vi "ReadPAQtags.vi"(8 "error in (no error)":errorcluster, 11 "DBAL-BIN in":refnum<class "DBAL-BIN.lvclass">) -> (0 "error out":errorcluster, 2 "PAQ_TAGs":T1 {"TAGprop"."TagFunc" format="%08x"; "TAGprop"."RangeL" format="%.2f"; "TAGprop"."RangeH" format="%.2f"}, 3 "DBAL-BIN out":refnum<class "DBAL-BIN.lvclass">)   [LabVIEW 2020, in "DBAL-BIN.lvclass"]
doc: "Read the PAQ Qtype TAG properties from the database"
uses:
  DBAL-BIN.lvclass
  controls/DBAL_TAGprops.ctl
  controls/DBAL_TAGpropEdit.ctl
  Common/controls/typedef_com_TagProp.ctl
  DBAL-BIN.lvclass/DBAL-BIN.ctl
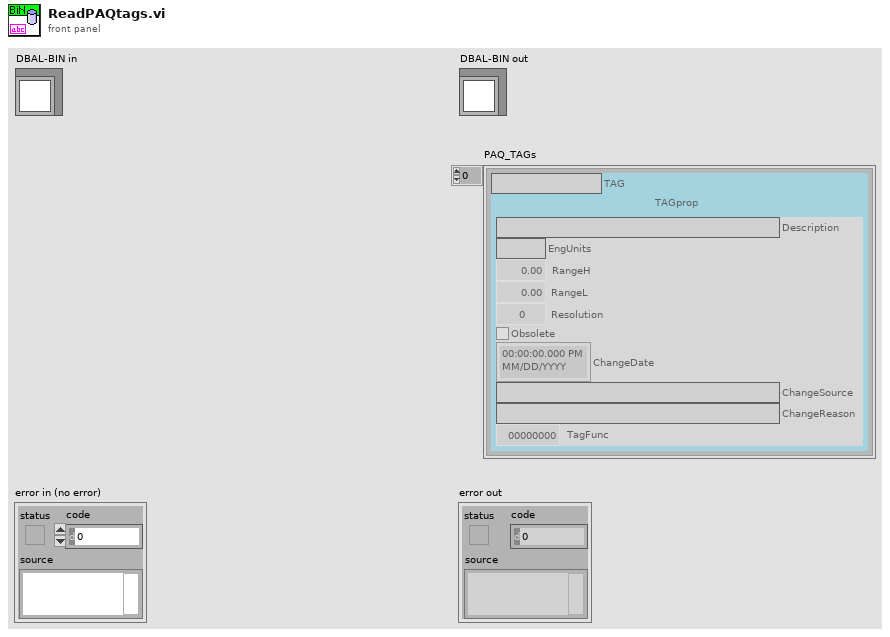
[diagram p1: front panel]
types:
  T1 = typedef "DBAL_TAGprops.ctl" = T2[]
  T2 = typedef "DBAL_TAGpropEdit.ctl" = cluster{"TAG":string, "TAGprop":T3}
  T3 = typedef "typedef_com_TagProp.ctl" = cluster{"Description":string, "EngUnits":string, "RangeH":dbl, "RangeL":dbl, "Resolution":i32, "Obsolete":bool, "ChangeDate":timestamp, "ChangeSource":string, "ChangeReason":string, "TagFunc":u32}
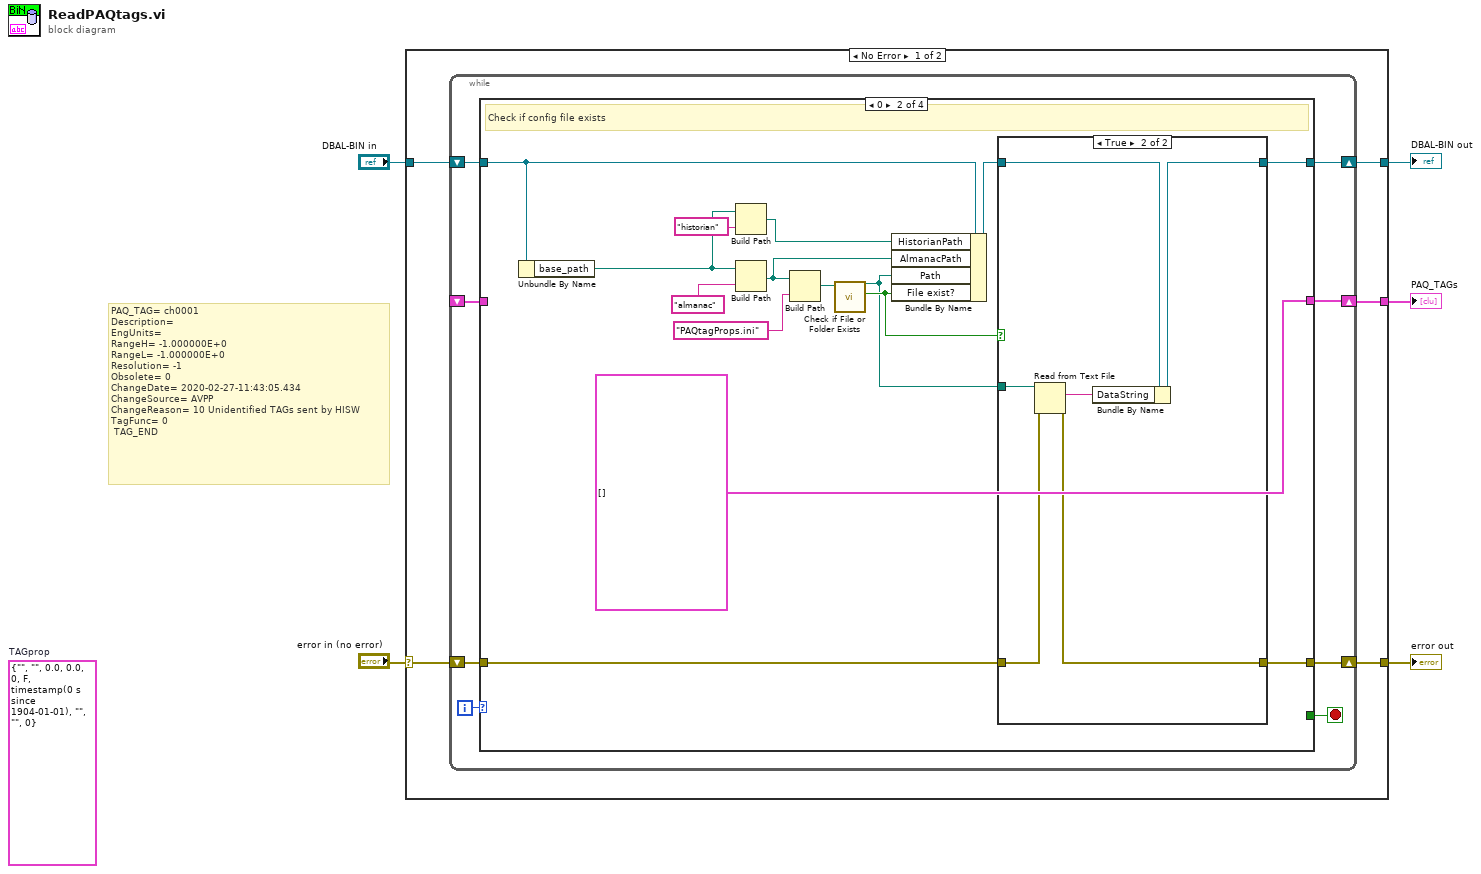
[diagram p0: block diagram]
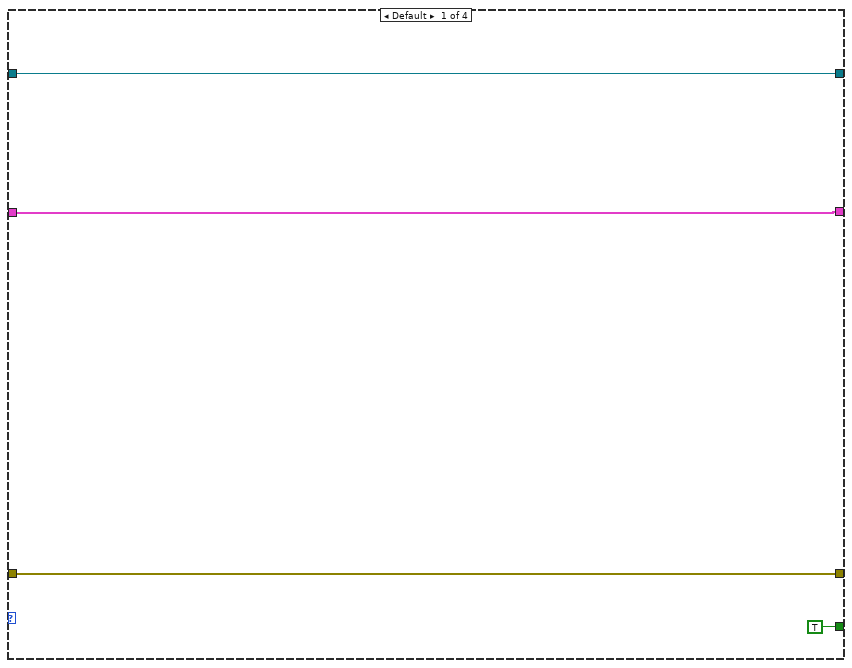
[diagram p2: hidden frame]
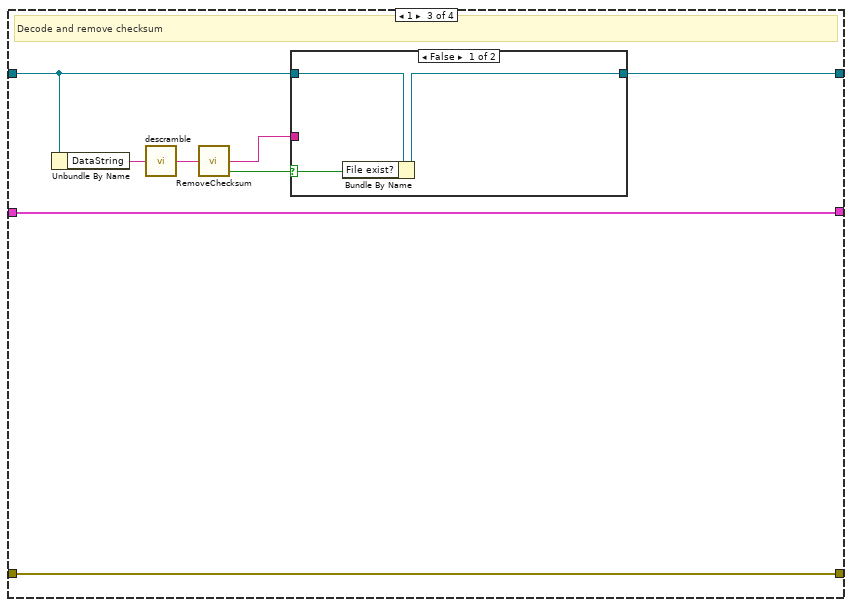
[diagram p4: hidden frame]
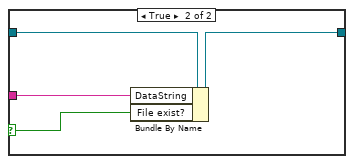
[diagram p5: hidden frame]
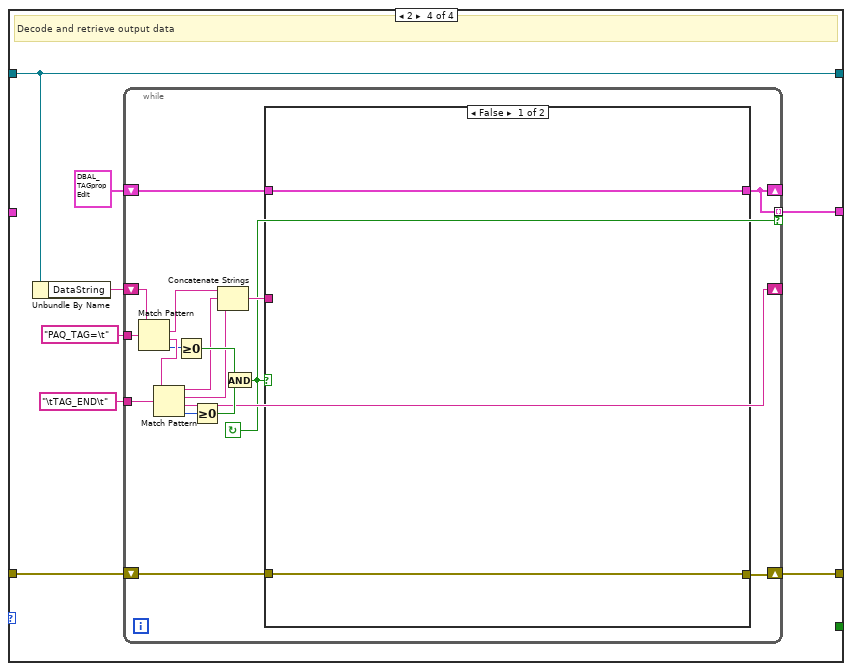
[diagram p6: hidden frame]
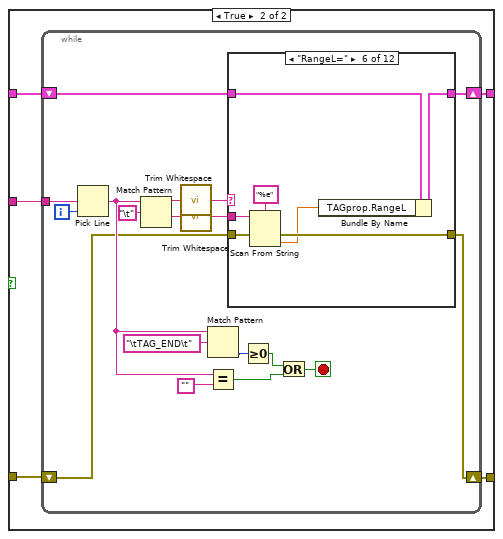
[diagram p7: hidden frame]
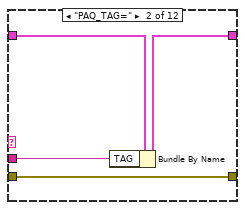
[diagram p9: hidden frame]
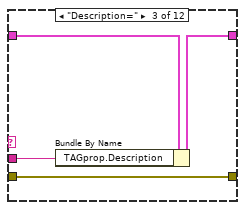
[diagram p10: hidden frame]
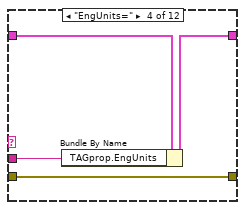
[diagram p11: hidden frame]
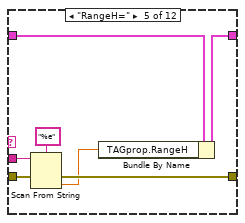
[diagram p12: hidden frame]
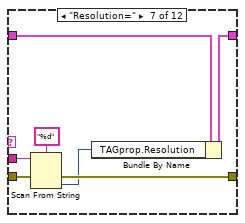
[diagram p13: hidden frame]
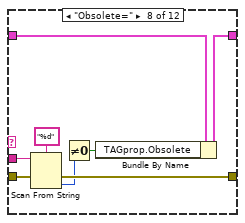
[diagram p14: hidden frame]
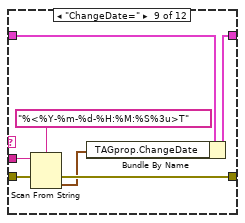
[diagram p15: hidden frame]
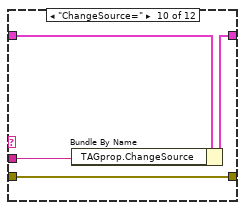
[diagram p16: hidden frame]
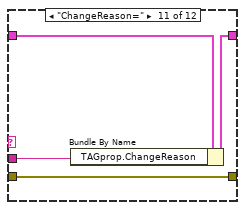
[diagram p17: hidden frame]
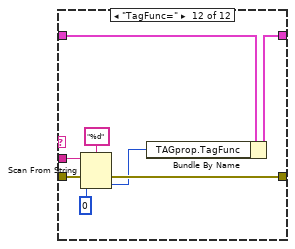
[diagram p18: hidden frame]
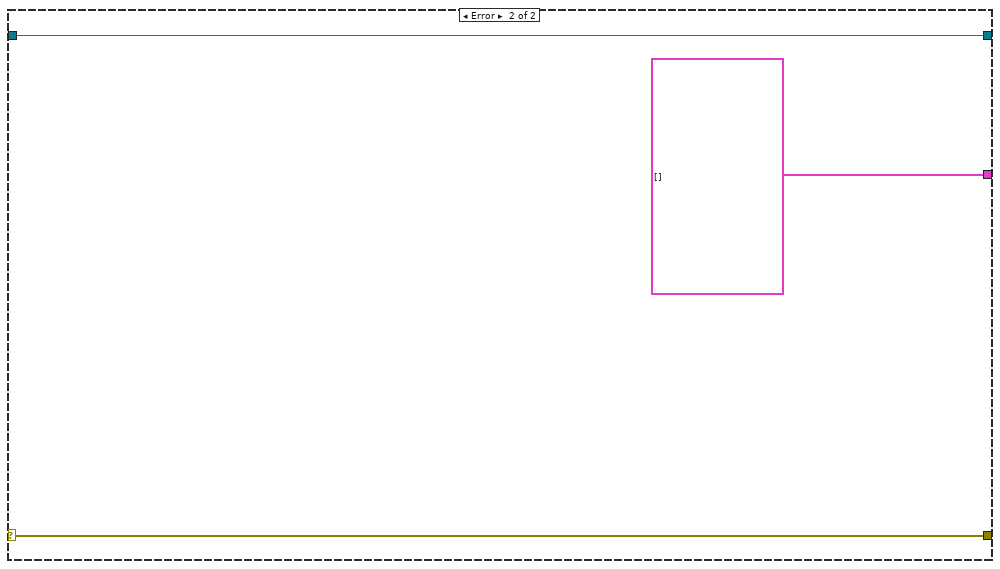
[diagram p19: hidden frame]
diagram:
  (unwired) T3 {"Description"="", "EngUnits"="", "RangeH"=0.0, "RangeL"=0.0, "Resolution"=0, "Obsolete"=FALSE, "ChangeDate"=timestamp(0 s since 1904-01-01), "ChangeSource"="", "ChangeReason"="", "TagFunc"=0}  # TAGprop
  # "PAQ_TAG=\tch0001\t\nDescription=\t\t\nEngUnits=\t\t\nRangeH=\t-1.000000E+0\t\nRangeL=\t-1.000000E+0\t\nResolution=\t-1\t\nObsolete=\t0\t\nChangeDate=\t2020-02-27-11:43:05.434\t\nChangeSource=\tAVPP\t\nChangeReason=\t10 Unidentified TAGs sent by HISW\t\nTagFunc=\t0\t\n\tTAG_END"
  n1 = case shown="No Error" "error in (no error)" {
    selector: "error in (no error)" -> [w10 w180]
    tunnel: "DBAL-BIN in" -> [w9 w178]
    tunnel: [w7 w180] -> w3
    tunnel: [w6 T1 [] ("PAQ_TAGs")] -> w2
    tunnel: [w8 w178] -> w1
    frame No Error {
      n2 = while {
        shift-right: [w13] -> w8
        shift-left: w9 -> [w14]
        shift-right: [w16] -> w7
        shift-left: w10 -> [w17]
        shift-right: [w12] -> w6
        shift-left: _ -> [w11]
        i -> [w18]
        stop <- w15 stop-if-true
        n3 = case shown="0" w18 {
          tunnel: w17 -> [w21 w35 w53 w63]
          tunnel: [w21 w34 w53 w62] -> w16
          tunnel: [TRUE _ _ _] -> w15
          tunnel: w14 -> [w20 w24 w51 w68]
          tunnel: [w20 w33 w50 w68] -> w13
          tunnel: [w19 T1 [] ("PAQ_TAGs") w46 w61] -> w12
          tunnel: w11 -> [w19 _ w46 _]
          frame Default {
          }
          frame 0 {
            # "Check if config file exists"
            n4 = Unbundle By Name(w24) -> ("base_path"=w23:path)
            n5 = Build Path(base path=w23, name or relative path="historian") -> (appended path=w25:path)
            n6 = Build Path(base path=w23, name or relative path="almanac") -> (appended path=w27:path)
            n7 = Build Path(base path=w27, name or relative path="PAQtagProps.ini") -> (appended path=w26:path)
            n8 = call <vilib>:"Check if File or Folder Exists.vi"("path"=w26) -> ("file or folder exists?"=w37:bool, "dup path"=w36:path)  [unwired: 8 in, 1 out]
            n9 = Bundle By Name(cluster=w24, "HistorianPath"=w25, "AlmanacPath"=w27, "Path"=w36, "File exist?"=w37) -> (w32:refnum<class "DBAL-BIN.lvclass">)
            n10 = case shown="True" w37 {
              tunnel: w36 -> [_ w43]
              tunnel: w35 -> [w39 w42]
              tunnel: [w39 w41] -> w34
              tunnel: [w38 w44] -> w33
              tunnel: w32 -> [w38 w45]
              frame False {
              }
              frame True {
                n11 = Read from Text File(file (use dialog)=w43, error in=w42) -> (text=w40:string, error out=w41:errorcluster)  [unwired: 2 in, 2 out]
                n12 = Bundle By Name(cluster=w45, "DataString"=w40) -> (w44:refnum<class "DBAL-BIN.lvclass">)
              }
            }
          }
          frame 1 {
            # "Decode and remove checksum"
            n13 = Unbundle By Name(w51) -> ("DataString"=w48:string)
            n14 = call "descramble.vi"("scrambled"=w48) -> ("OUT"=w47:string)  [unwired: 6 in]
            n15 = call "RemoveChecksum.vi"("IN"=w47) -> ("Check OK?"=w52:bool, "OUT"=w49:string)  [unwired: 3 in]
            n16 = case shown="False" w52 {
              selector: w52 -> [w56 w57]
              tunnel: w51 -> [w55 w60]
              tunnel: [w54 w58] -> w50
              tunnel: w49 -> [_ w59]
              frame False {
                n17 = Bundle By Name(cluster=w55, "File exist?"=w56) -> (w54:refnum<class "DBAL-BIN.lvclass">)
              }
              frame True {
                n18 = Bundle By Name(cluster=w60, "DataString"=w59, "File exist?"=w57) -> (w58:refnum<class "DBAL-BIN.lvclass">)
              }
            }
          }
          frame 2 {
            # "Decode and retrieve output data"
            n19 = Unbundle By Name(w68) -> ("DataString"=w67:string)
            n20 = while {
              shift-right: [w77] -> _
              shift-left: w67 -> [w86]
              tunnel: "PAQ_TAG=\t" -> [w85]
              tunnel: "\tTAG_END\t" -> [w83]
              shift-right: [w76] -> _
              shift-left: T2 {"TAG"="", "TAGprop"={"Description"="", "EngUnits"="", "RangeH"=0.0, "RangeL"=0.0, "Resolution"=0, "Obsolete"=FALSE, "ChangeDate"=timestamp(0 s since 1904-01-01), "ChangeSource"="", "ChangeReason"="", "TagFunc"=0}} ("TAGpropertyEdit") -> [w78]
              tunnel: [w76] -> w61 mode=indexing if=w69
              shift-right: [w70] -> w62
              shift-left: w63 -> [w71]
              stop <- w69 continue-if-true
              n21 = Match Pattern(string=w86, regular expression=w85) -> (match substring=w75:string, after substring=w84:string, offset past match=w82:i32)  [unwired: 1 in, 1 out]
              n22 = Match Pattern(string=w84, regular expression=w83) -> (before substring=w74:string, match substring=w73:string, after substring=w77:string, offset past match=w81:i32)  [unwired: 1 in]
              n23 = Greater Or Equal To 0?(x=w82) -> (x >= 0?=w80:bool)
              n24 = Greater Or Equal To 0?(x=w81) -> (x >= 0?=w79:bool)
              n25 = Concatenate Strings(w75, w74, w73) -> (w72:string)
              n26 = And(x=w80, y=w79) -> (x .and. y?=w69:bool)
              n27 = case shown="False" w69 {
                tunnel: w78 -> [w88 w92]
                tunnel: [w88 w91] -> w76
                tunnel: w72 -> [_ w93]
                tunnel: w71 -> [w87 w90]
                tunnel: [w87 w89] -> w70
                frame False {
                }
                frame True {
                  n28 = while {
                    tunnel: w93 -> [w94]
                    shift-right: [w99] -> w91
                    shift-left: w92 -> [w100]
                    shift-right: [w95] -> w89
                    shift-left: w90 -> [w96]
                    i -> [w111]
                    stop <- w105 stop-if-true
                    n29 = Pick Line(multi-line string=w94, line index=w111) -> (output string=w104:string)  [unwired: 1 in]
                    n30 = Match Pattern(string=w104, regular expression="\t") -> (before substring=w102:string, after substring=w98:string)  [unwired: 1 in, 2 out]
                    n31 = call <vilib>:"Trim Whitespace.vi"("string"=w102) -> ("trimmed string"=w101:string)  [unwired: 1 in]
                    n32 = call <vilib>:"Trim Whitespace.vi"("string"=w98) -> ("trimmed string"=w97:string)  [unwired: 1 in]
                    n33 = Match Pattern(string=w104, regular expression="\tTAG_END\t") -> (offset past match=w108:i32)  [unwired: 1 in, 3 out]
                    n34 = Equal?(x=w104, y="") -> (x = y?=w106:bool)
                    n35 = case shown="\"RangeL=\"" w101 {
                      tunnel: w100 -> [w113 w117 w121 w125 w132 w139 w146 w154 w161 w165 w169 w177]
                      tunnel: [w113 w116 w120 w124 w131 w138 w145 w153 w160 w164 w168 w176] -> w99
                      tunnel: w97 -> [_ w115 w119 w123 w129 w136 w143 w151 w159 w162 w166 w174]
                      tunnel: w96 -> [w112 w114 w118 w122 w128 w135 w142 w150 w158 w163 w167 w173]
                      tunnel: [w112 w114 w118 w122 w127 w134 w141 w149 w157 w163 w167 w172] -> w95
                      frame Default {
                      }
                      frame "PAQ_TAG=" {
                        n36 = Bundle By Name(cluster=w117, "TAG"=w115) -> (w116:T2)
                      }
                      frame "Description=" {
                        n37 = Bundle By Name(cluster=w121, "TAGprop.Description"=w119) -> (w120:T2)
                      }
                      frame "EngUnits=" {
                        n38 = Bundle By Name(cluster=w125, "TAGprop.EngUnits"=w123) -> (w124:T2)
                      }
                      frame "RangeH=" {
                        n39 = Scan From String(format string="%e", input string=w129, error in=w128) -> (error out=w127:errorcluster, output 1=w126:dbl)  [unwired: 2 in, 2 out]
                        n40 = Bundle By Name(cluster=w132, "TAGprop.RangeH"=w126) -> (w131:T2)
                      }
                      frame "RangeL=" {
                        n41 = Scan From String(format string="%e", input string=w136, error in=w135) -> (error out=w134:errorcluster, output 1=w133:dbl)  [unwired: 2 in, 2 out]
                        n42 = Bundle By Name(cluster=w139, "TAGprop.RangeL"=w133) -> (w138:T2)
                      }
                      frame "Resolution=" {
                        n43 = Scan From String(format string="%d", input string=w143, error in=w142) -> (error out=w141:errorcluster, output 1=w140:i32)  [unwired: 2 in, 2 out]
                        n44 = Bundle By Name(cluster=w146, "TAGprop.Resolution"=w140) -> (w145:T2)
                      }
                      frame "Obsolete=" {
                        n45 = Scan From String(format string="%d", input string=w151, error in=w150) -> (error out=w149:errorcluster, output 1=w148:i32)  [unwired: 2 in, 2 out]
                        n46 = Not Equal To 0?(x=w148) -> (x != 0?=w147:bool)
                        n47 = Bundle By Name(cluster=w154, "TAGprop.Obsolete"=w147) -> (w153:T2)
                      }
                      frame "ChangeDate=" {
                        n48 = Scan From String(format string="%<%Y-%m-%d-%H:%M:%S%3u>T", input string=w159, error in=w158) -> (error out=w157:errorcluster, output 1=w155:timestamp)  [unwired: 2 in, 2 out]
                        n49 = Bundle By Name(cluster=w161, "TAGprop.ChangeDate"=w155) -> (w160:T2)
                      }
                      frame "ChangeSource=" {
                        n50 = Bundle By Name(cluster=w165, "TAGprop.ChangeSource"=w162) -> (w164:T2)
                      }
                      frame "ChangeReason=" {
                        n51 = Bundle By Name(cluster=w169, "TAGprop.ChangeReason"=w166) -> (w168:T2)
                      }
                      frame "TagFunc=" {
                        n52 = Scan From String(format string="%d", input string=w174, error in=w173, default 1=u32 0 ("default value 1")) -> (error out=w172:errorcluster, output 1=w171:u32)  [unwired: 1 in, 2 out]
                        n53 = Bundle By Name(cluster=w177, "TAGprop.TagFunc"=w171) -> (w176:T2)
                      }
                    }
                    n54 = Greater Or Equal To 0?(x=w108) -> (x >= 0?=w107:bool)
                    n55 = Or(x=w107, y=w106) -> (x .or. y?=w105:bool)
                  }
                }
              }
            }
          }
        }
      }
    }
    frame Error {
    }
  }
  "error out" <- w3
  "DBAL-BIN out" <- w1
  "PAQ_TAGs" <- w2
